vi "Facade 1.vi"(0 "Data In":T4 caption="数据输入", 2 "Display State In":T2 caption="显示状态输入", 3 "Container State":T3 caption="容器状态") -> (6 "Data Out":T4 caption="数据输出", 7 "Display State Out":T2 caption="显示状态输出", 8 "Action":T1 caption="动作")   [LabVIEW 2011, in "XSuperLink.xctl"]
uses:
  XSuperLink.xctl
  Data 1.ctl
  <vilib>/_xctls/Container State.ctl
  State 1.ctl
  <vilib>/_xctls/Action.ctl
  <vilib>/Platform/browser.llb/Open URL in Default Browser (string).vi
  <vilib>/_xctls/XControlSupport.lvlib
panel:
  out "link":bool
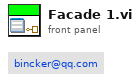
[diagram p1: front panel]
types:
  T1 = typedef "XControlSupport.lvlib/Action.ctl" = cluster{"Data Changed?":bool, "State Changed?":bool, "Action Name":string}
  T2 = typedef "XSuperLink.xctl/State 1.ctl" = cluster{"Accept":bool, "link":string}
  T3 = typedef "XControlSupport.lvlib/Container State.ctl" = cluster{"Indicator?":bool, "Run Mode?":bool, " Refnum":refnum<vi>}
  T4 = typedef "XSuperLink.xctl/Data 1.ctl" = string
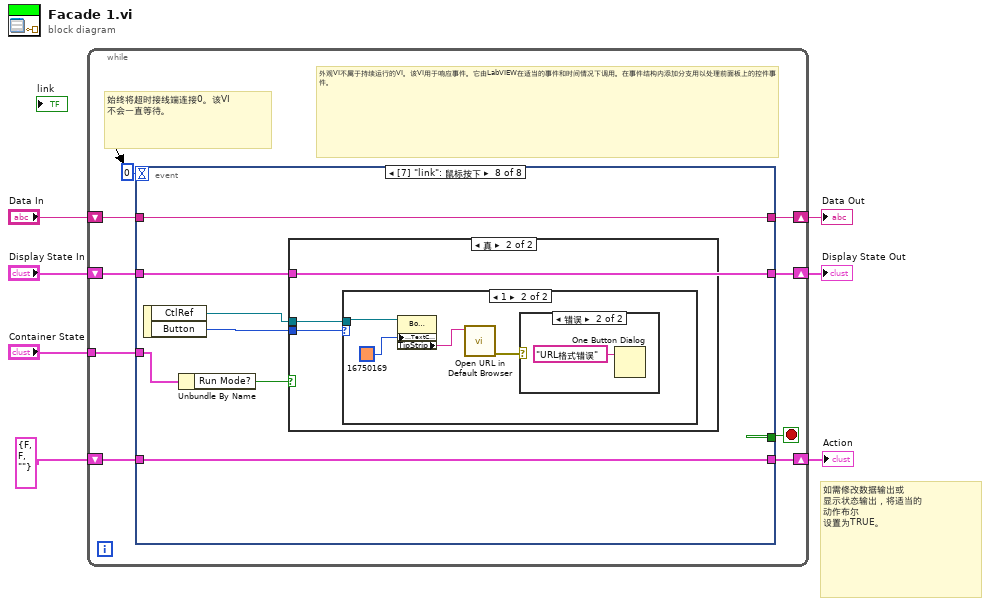
[diagram p0: block diagram]
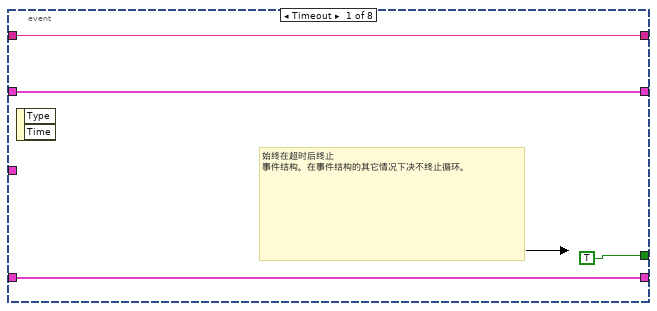
[diagram p2: hidden frame]
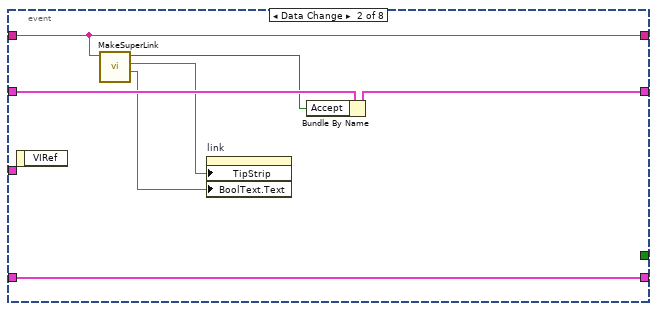
[diagram p3: hidden frame]
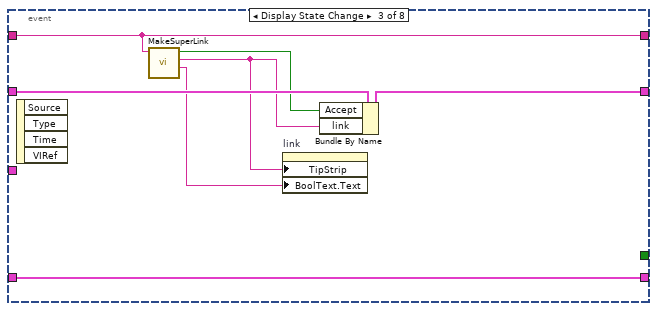
[diagram p4: hidden frame]
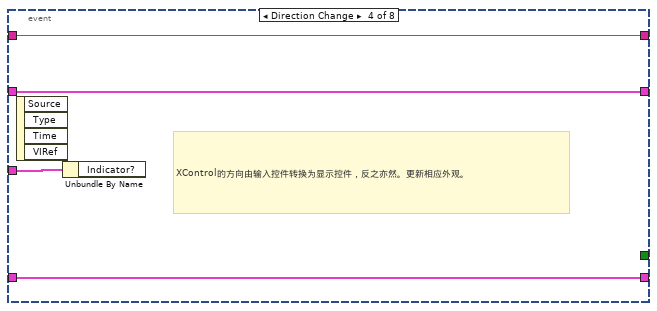
[diagram p5: hidden frame]
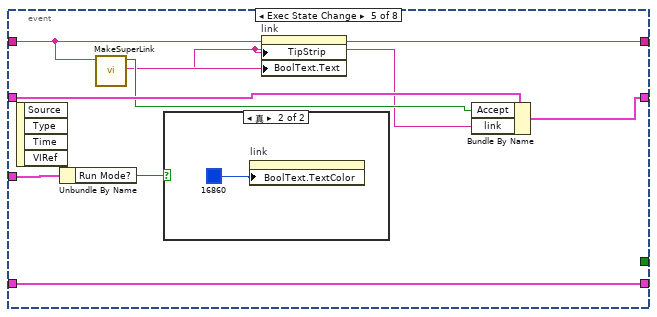
[diagram p6: hidden frame]
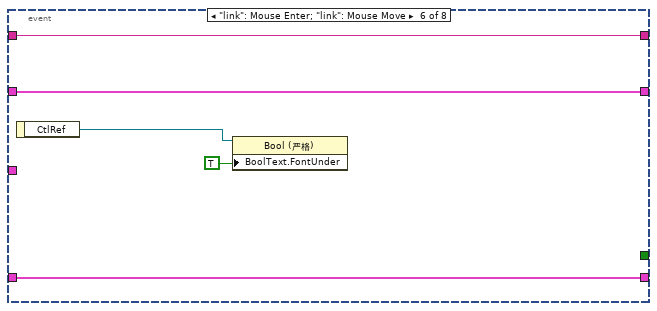
[diagram p8: hidden frame]
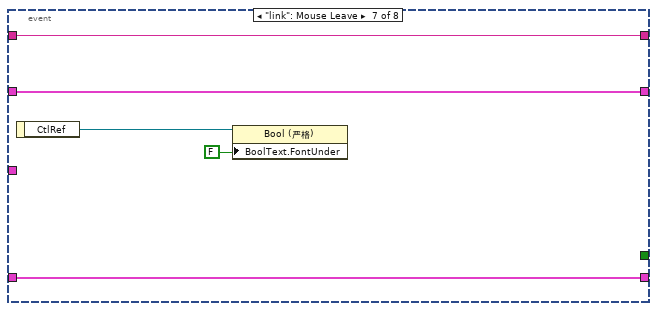
[diagram p9: hidden frame]
diagram:
  # "如需修改数据输出或\n显示状态输出，将适当的\n动作布尔\n设置为TRUE。"
  n1 = while {
    shift-right: [w15] -> w4
    shift-left: "Display State In" -> [w16]
    tunnel: "Container State" -> [w12]
    shift-right: [w10] -> w7
    shift-left: "Data In" -> [w11]
    shift-right: [w8] -> w2
    shift-left: T1 {"Data Changed?"=FALSE, "State Changed?"=FALSE, "Action Name"=""} ("Action") -> [w9]
    stop <- w14 stop-if-true
    # "外观VI不属于持续运行的VI。该VI用于响应事件。它由LabVIEW在适当的事件和时间情况下调用。在事件结构内添加分支用以处理前面板上的控件事件。"
    # "始终将超时接线端连接0。该VI\n不会一直等待。"
    n2 = event shown="[7] \"link\": 鼠标按下" {
      selector: _ -> [_ _ _ _ _ _ _ _]
      dyn-events: _ -> [_ _ _ _ _ _ _ _]
      timeout: 0 -> [_ _ _ _ _ _ _ _]
      tunnel: w16 -> [w18 w26 w34 w37 w44 w50 w55 w60]
      tunnel: [w18 w25 w32 w37 w43 w50 w55 w60] -> w15
      tunnel: [TRUE _ _ _ _ _ _ _] -> w14
      tunnel: w12 -> [_ _ _ w38 w47 _ _ w62]
      tunnel: w11 -> [w17 w22 w29 w36 w40 w52 w57 w59]
      tunnel: [w17 w22 w29 w36 w40 w52 w57 w59] -> w10
      tunnel: [w19 w27 w33 w35 w46 w53 w58 w63] -> w8
      tunnel: w9 -> [w19 w27 w33 w35 w46 w53 w58 w63]
      event Timeout {
        # "始终在超时后终止\n事件结构。在事件结构的其它情况下决不终止循环。"
        n3 = event-data() -> ()  [unwired: 1 in, 2 out]
      }
      event Data Change {
        n4 = event-data() -> ()  [unwired: 1 in, 1 out]
        n5 = call "MakeSuperLink.vi"("data"=w22) -> ("show info"=w23:string, "superlinkStr"=w21:string, "Accept"=w24:bool)  [unwired: 8 in]
        n6 = property on="link" class="Bool (严格)"("TipStrip"=w21, "BoolText.Text"=w23) -> ()  [unwired: 2 in, 2 out]
        n7 = Bundle By Name(cluster=w26, "Accept"=w24) -> (w25:T2)
      }
      event Display State Change {
        n8 = event-data() -> ()  [unwired: 1 in, 4 out]
        n9 = call "MakeSuperLink.vi"("data"=w29) -> ("show info"=w30:string, "superlinkStr"=w28:string, "Accept"=w31:bool)  [unwired: 8 in]
        n10 = property on="link" class="Bool (严格)"("TipStrip"=w28, "BoolText.Text"=w30) -> ()  [unwired: 2 in, 2 out]
        n11 = Bundle By Name(cluster=w34, "Accept"=w31, "link"=w28) -> (w32:T2)
      }
      event Direction Change {
        # "XControl的方向由输入控件转换为显示控件，反之亦然。更新相应外观。"
        n12 = event-data() -> ()  [unwired: 1 in, 4 out]
        n13 = Unbundle By Name(w38) -> ()  [unwired: 1 out]
      }
      event Exec State Change {
        n14 = event-data() -> ()  [unwired: 1 in, 4 out]
        n15 = Unbundle By Name(w47) -> ("Run Mode?"=w45:bool)
        n16 = call "MakeSuperLink.vi"("data"=w40) -> ("show info"=w41:string, "superlinkStr"=w39:string, "Accept"=w42:bool)  [unwired: 8 in]
        n17 = case shown="真" w45 {
          frame False {
          }
          frame True {
            n18 = property on="link" class="Bool (严格)"("BoolText.TextColor"=u32 16860) -> ()  [unwired: 2 in, 2 out]
          }
        }
        n19 = property on="link" class="Bool (严格)"("TipStrip"=w39, "BoolText.Text"=w41) -> ()  [unwired: 2 in, 2 out]
        n20 = Bundle By Name(cluster=w44, "Accept"=w42, "link"=w39) -> (w43:T2)
      }
      event "link": Mouse Enter; "link": Mouse Move {
        n21 = event-data() -> ("CtlRef"=w51:refnum<vi>)  [unwired: 1 in]
        n22 = property class="Bool (严格)"(reference=w51, "BoolText.FontUnder"=TRUE ("布尔文本.字体:下划线")) -> ()  [unwired: 1 in, 2 out]
      }
      event "link": Mouse Leave {
        n23 = event-data() -> ("CtlRef"=w56:refnum<vi>)  [unwired: 1 in]
        n24 = property class="Bool (严格)"(reference=w56, "BoolText.FontUnder"=FALSE ("布尔文本.字体:下划线")) -> ()  [unwired: 1 in, 2 out]
      }
      event "link": Mouse Down {
        n25 = event-data() -> ("CtlRef"=w64:refnum<vi>, "Button"=w65:u16)  [unwired: 1 in]
        n26 = Unbundle By Name(w62) -> ("Run Mode?"=w61:bool)
        n27 = case shown="真" w61 {
          tunnel: w65 -> [_ w67]
          tunnel: w64 -> [_ w66]
          tunnel: w60 -> [_ _]
          frame False {
          }
          frame True {
            n28 = case shown="1" w67 {
              tunnel: w66 -> [_ w71]
              frame 0, Default {
              }
              frame 1 {
                n29 = property class="Bool (严格)"(reference=w71, "BoolText.TextColor"=u32 16750169) -> ("TipStrip"=w68:string)  [unwired: 1 in, 2 out]
                n30 = call-poly <vilib>:"Open URL in Default Browser.vi"("URL"=w68) -> ("error out"=w69:errorcluster)  [unwired: 5 in, 1 out]
                n31 = case shown="错误" w69 {
                  frame No Error {
                  }
                  frame Error {
                    n32 = One Button Dialog(message="URL格式错误" ("消息")) -> ()  [unwired: 1 in, 1 out]
                  }
                }
              }
            }
          }
        }
      }
    }
  }
  "Display State Out" <- w4
  "Data Out" <- w7
  "Action" <- w2
